vi "um... Prototype 1.vi"() -> ()   [LabVIEW 2014]
uses:
  SRE Enum.ctl
  Support Code/Robot Global Data.vi
panel:
  in  "Sequence":T1(ring)
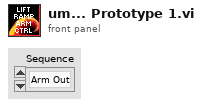
[diagram p1: front panel]
types:
  T1 = enum16{"Arm Out", "All In", "Lift Down", "Ramp Out"}
  T2 = typedef "SRE Enum.ctl" = enum16{"Start", "Run", "End"}
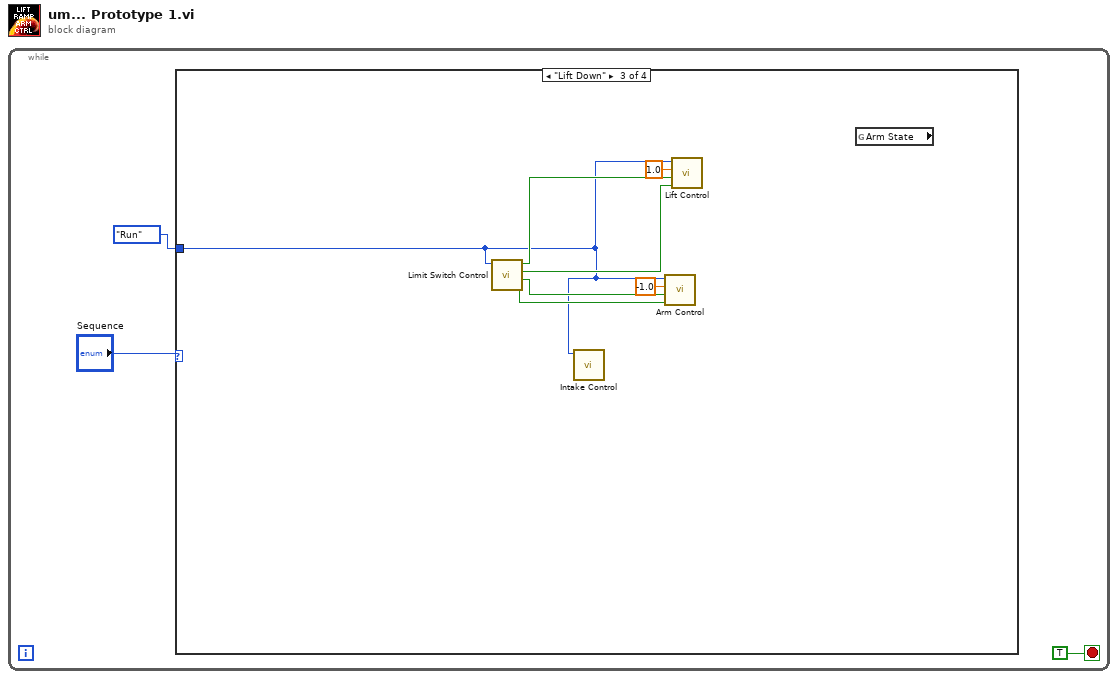
[diagram p0: block diagram]
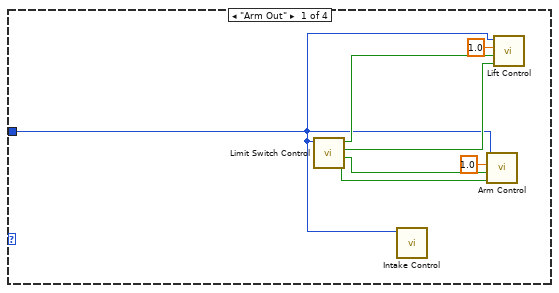
[diagram p2: hidden frame]
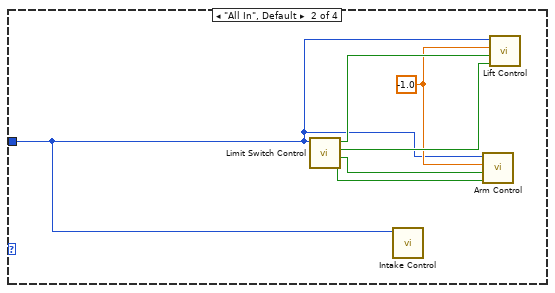
[diagram p3: hidden frame]
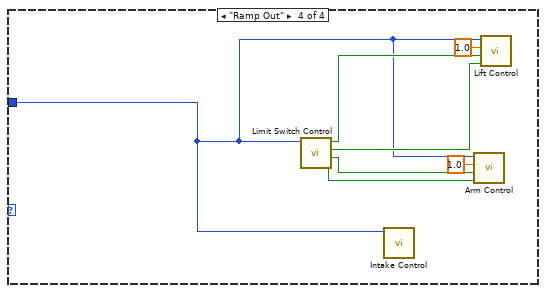
[diagram p4: hidden frame]
diagram:
  n1 = while {
    stop <- TRUE stop-if-true
    n2 = case shown="\"Lift Down\"" "Sequence" {
      tunnel: SRE_Enum."Run" ("Run Mode") -> [w4 w11 w19 w26]
      frame "Arm Out" {
        n3 = call "Limit Switch Control.vi"("Run Mode"=w4) -> ("Arm Bottom"=w8:bool, "Arm Top"=w7:bool, "Lift Bottom"=w10:bool, "Lift Top"=w9:bool)  [unwired: 7 in]
        n4 = call "Intake Control.vi"("Enum"=w4) -> ()  [unwired: 11 in]
        n5 = call "Arm Control.vi"("bottom"=w8, "top"=w7, "Motor"=1.0, "Enum"=w4) -> ()  [unwired: 7 in, 1 out]
        n6 = call "Lift Control.vi"("bottom"=w10, "top"=w9, "Motor"=1.0, "Enum"=w4) -> ()  [unwired: 7 in, 1 out]
      }
      frame "All In", Default {
        w12 = -1.0
        n7 = call "Limit Switch Control.vi"("Run Mode"=w11) -> ("Arm Bottom"=w15:bool, "Arm Top"=w16:bool, "Lift Bottom"=w13:bool, "Lift Top"=w14:bool)  [unwired: 7 in]
        n8 = call "Intake Control.vi"("Enum"=w11) -> ()  [unwired: 11 in]
        n9 = call "Arm Control.vi"("bottom"=w15, "top"=w16, "Motor"=w12, "Enum"=w11) -> ()  [unwired: 7 in, 1 out]
        n10 = call "Lift Control.vi"("bottom"=w13, "top"=w14, "Motor"=w12, "Enum"=w11) -> ()  [unwired: 7 in, 1 out]
      }
      frame "Lift Down" {
        n11 = call "Limit Switch Control.vi"("Run Mode"=w19) -> ("Arm Bottom"=w21:bool, "Arm Top"=w20:bool, "Lift Bottom"=w23:bool, "Lift Top"=w22:bool)  [unwired: 7 in]
        n12 = call "Intake Control.vi"("Enum"=w19) -> ()  [unwired: 11 in]
        n13 = call "Arm Control.vi"("bottom"=w21, "top"=w20, "Motor"=-1.0, "Enum"=w19) -> ()  [unwired: 7 in, 1 out]
        n14 = call "Lift Control.vi"("bottom"=w23, "top"=w22, "Motor"=1.0, "Enum"=w19) -> ()  [unwired: 7 in, 1 out]
        n15 = global read "Robot Global Data.vi" "Arm State"() -> ()  [unwired: 1 out]
      }
      frame "Ramp Out" {
        n16 = call "Limit Switch Control.vi"("Run Mode"=w26) -> ("Arm Bottom"=w28:bool, "Arm Top"=w27:bool, "Lift Bottom"=w30:bool, "Lift Top"=w29:bool)  [unwired: 7 in]
        n17 = call "Intake Control.vi"("Enum"=w26) -> ()  [unwired: 11 in]
        n18 = call "Arm Control.vi"("bottom"=w28, "top"=w27, "Motor"=1.0, "Enum"=w26) -> ()  [unwired: 7 in, 1 out]
        n19 = call "Lift Control.vi"("bottom"=w30, "top"=w29, "Motor"=1.0, "Enum"=w26) -> ()  [unwired: 7 in, 1 out]
      }
    }
  }
